vi "Elevator Control PID.vi"(8 "Settings":T2={"output range"={"output high"=1.0, "output low"=-0.75}, "min speed"=0.05, "homing speed"=0.05, "Position Max"=60.0, "PIDF gains"={"Kp"=0.2, "Ki"=0.0, "Kd"=0.2, "Kf"=0.0}, "gravity"=0.05, "Rate Limit in/sec"=30.0} {"Rate Limit in/sec" format="%#_13g"; "gravity" format="%#_13g"; "PIDF gains"."Kf" format="%.5f"; "PIDF gains"."Kd" format="%.3f"; "PIDF gains"."Ki" format="%.3f"; "PIDF gains"."Kp" format="%.3f"; "Position Max" format="%#_13g"; "homing speed" format="%#_13g"; "min speed" format="%#_13g"; "output range"."output low" format="%.2f"; "output range"."output high" format="%.2f"}, 9 "Manual":bool, 10 "Setpoint":dbl, 11 "Controller In":T3={"Setpoint"=0.0, "Output"=0.0, "DriveMotor1"={"DeviceStatus"={"status"=FALSE, "code"=0, "source"=""}, "Type"=enum."PWM", "PWM"={"PWM Channel"=enum."Invalid", "DeadBand"={"Name"="", "maxPositivePwm"=0, "minPositivePwm"=0, "centerPwm"=0, "maxNegativePwm"=0, "minNegativePwm"=0, "angularRange"=0}}, "CAN"={"Device Number"=0, "SetOutput VI Ref"=variant(enum8{"Percent VBus", "Current", "Speed", "Position", "Voltage"} enum."Percent VBus"), "GetOutput VI Ref"=variant(refnum<k1> refnum), "Enable VI Ref"=variant(dbl 12.0), "Disable VI Ref"=variant(enum8{"Percent VBus", "Speed", "Position", "Slave", "Unchanged / Invalid"} enum."Percent VBus"), "Data"=variant(enum16{"Controller 1"} enum."Controller 1")}, "Invert"=FALSE, "DIO PWM"={"PWM \"Enable\" Channel"=enum."Invalid", "DIOChannel"=enum."Invalid", "PWM Rate"=0.0}}, "Encoder"={"DevStatus"={"status"=FALSE, "code"=0, "source"=""}, "EncoderIndex"=enum."Invalid", "CounterIndex"=enum."Invalid", "DistancePerCount"=1.0, "Decoding Type"=enum."4x"}, "DriveMotor2"={"DeviceStatus"={"status"=FALSE, "code"=0, "source"=""}, "Type"=enum."PWM", "PWM"={"PWM Channel"=enum."Invalid", "DeadBand"={"Name"="", "maxPositivePwm"=0, "minPositivePwm"=0, "centerPwm"=0, "maxNegativePwm"=0, "minNegativePwm"=0, "angularRange"=0}}, "CAN"={"Device Number"=0, "SetOutput VI Ref"=variant(enum8{"Percent VBus", "Current", "Speed", "Position", "Voltage"} enum."Percent VBus"), "GetOutput VI Ref"=variant(refnum<k1> refnum), "Enable VI Ref"=variant(dbl 12.0), "Disable VI Ref"=variant(enum8{"Percent VBus", "Speed", "Position", "Slave", "Unchanged / Invalid"} enum."Percent VBus"), "Data"=variant(enum16{"Controller 1"} enum."Controller 1")}, "Invert"=FALSE, "DIO PWM"={"PWM \"Enable\" Channel"=enum."Invalid", "DIOChannel"=enum."Invalid", "PWM Rate"=0.0}}, "Top SW"={"DevStatus"={"status"=FALSE, "code"=0, "source"=""}, "DIO Channel"=enum."Invalid"}, "Bottom SW"={"DevStatus"={"status"=FALSE, "code"=0, "source"=""}, "DIO Channel"=enum."Invalid"}, "Is Done Moving?"=FALSE}) -> (0 "Switches":T1, 1 "PID is Done?":bool, 2 "Graph Out":T14(graph), 3 "Controller out":T3={"Setpoint"=0.0, "Output"=0.0, "DriveMotor1"={"DeviceStatus"={"status"=FALSE, "code"=0, "source"=""}, "Type"=enum."PWM", "PWM"={"PWM Channel"=enum."Invalid", "DeadBand"={"Name"="", "maxPositivePwm"=0, "minPositivePwm"=0, "centerPwm"=0, "maxNegativePwm"=0, "minNegativePwm"=0, "angularRange"=0}}, "CAN"={"Device Number"=0, "SetOutput VI Ref"=variant(enum8{"Percent VBus", "Current", "Speed", "Position", "Voltage"} enum."Percent VBus"), "GetOutput VI Ref"=variant(refnum<k1> refnum), "Enable VI Ref"=variant(dbl 12.0), "Disable VI Ref"=variant(enum8{"Percent VBus", "Speed", "Position", "Slave", "Unchanged / Invalid"} enum."Percent VBus"), "Data"=variant(enum16{"Controller 1"} enum."Controller 1")}, "Invert"=FALSE, "DIO PWM"={"PWM \"Enable\" Channel"=enum."Invalid", "DIOChannel"=enum."Invalid", "PWM Rate"=0.0}}, "Encoder"={"DevStatus"={"status"=FALSE, "code"=0, "source"=""}, "EncoderIndex"=enum."Invalid", "CounterIndex"=enum."Invalid", "DistancePerCount"=1.0, "Decoding Type"=enum."4x"}, "DriveMotor2"={"DeviceStatus"={"status"=FALSE, "code"=0, "source"=""}, "Type"=enum."PWM", "PWM"={"PWM Channel"=enum."Invalid", "DeadBand"={"Name"="", "maxPositivePwm"=0, "minPositivePwm"=0, "centerPwm"=0, "maxNegativePwm"=0, "minNegativePwm"=0, "angularRange"=0}}, "CAN"={"Device Number"=0, "SetOutput VI Ref"=variant(enum8{"Percent VBus", "Current", "Speed", "Position", "Voltage"} enum."Percent VBus"), "GetOutput VI Ref"=variant(refnum<k1> refnum), "Enable VI Ref"=variant(dbl 12.0), "Disable VI Ref"=variant(enum8{"Percent VBus", "Speed", "Position", "Slave", "Unchanged / Invalid"} enum."Percent VBus"), "Data"=variant(enum16{"Controller 1"} enum."Controller 1")}, "Invert"=FALSE, "DIO PWM"={"PWM \"Enable\" Channel"=enum."Invalid", "DIOChannel"=enum."Invalid", "PWM Rate"=0.0}}, "Top SW"={"DevStatus"={"status"=FALSE, "code"=0, "source"=""}, "DIO Channel"=enum."Invalid"}, "Bottom SW"={"DevStatus"={"status"=FALSE, "code"=0, "source"=""}, "DIO Channel"=enum."Invalid"}, "Is Done Moving?"=FALSE})   [LabVIEW 2017]
uses:
  Typedef/Controller Data.ctl
  <vilib>/Rock Robotics/WPI/MotorControl/WPI_MotorControlDeviceRef.ctl
  <vilib>/Rock Robotics/WPI/MotorControl/WPI_MotorControlType.ctl
  <vilib>/Rock Robotics/SystemInterfaces/DIO/FPGA_DIOPWMChannel.ctl
  <vilib>/Rock Robotics/WPI/PWM/WPI_PWMDeadband.ctl
  <vilib>/Rock Robotics/SystemInterfaces/DIO/FPGA_DIOChannel.ctl
  <vilib>/Rock Robotics/WPI/Encoder/WPI_EncoderDevRef.ctl
  <vilib>/Rock Robotics/SystemInterfaces/Encoder/FPGA_EncoderIdx.ctl
  <vilib>/Rock Robotics/SystemInterfaces/Counter/FPGA_CounterCtrSystemIndex.ctl
  <vilib>/Rock Robotics/WPI/Encoder/WPI_EncoderType.ctl
  <vilib>/Rock Robotics/WPI/DigitalInput/WPI_DigitalInputDevRef.ctl
  Typedef/Elevator Settings.ctl
  Implementation/Elevator Position Global.vi
  <vilib>/addons/control/pid/pid.llb/PID Output Rate Limiter (DBL).vi
  <vilib>/addons/control/pid/NI_PID_pid.lvlib
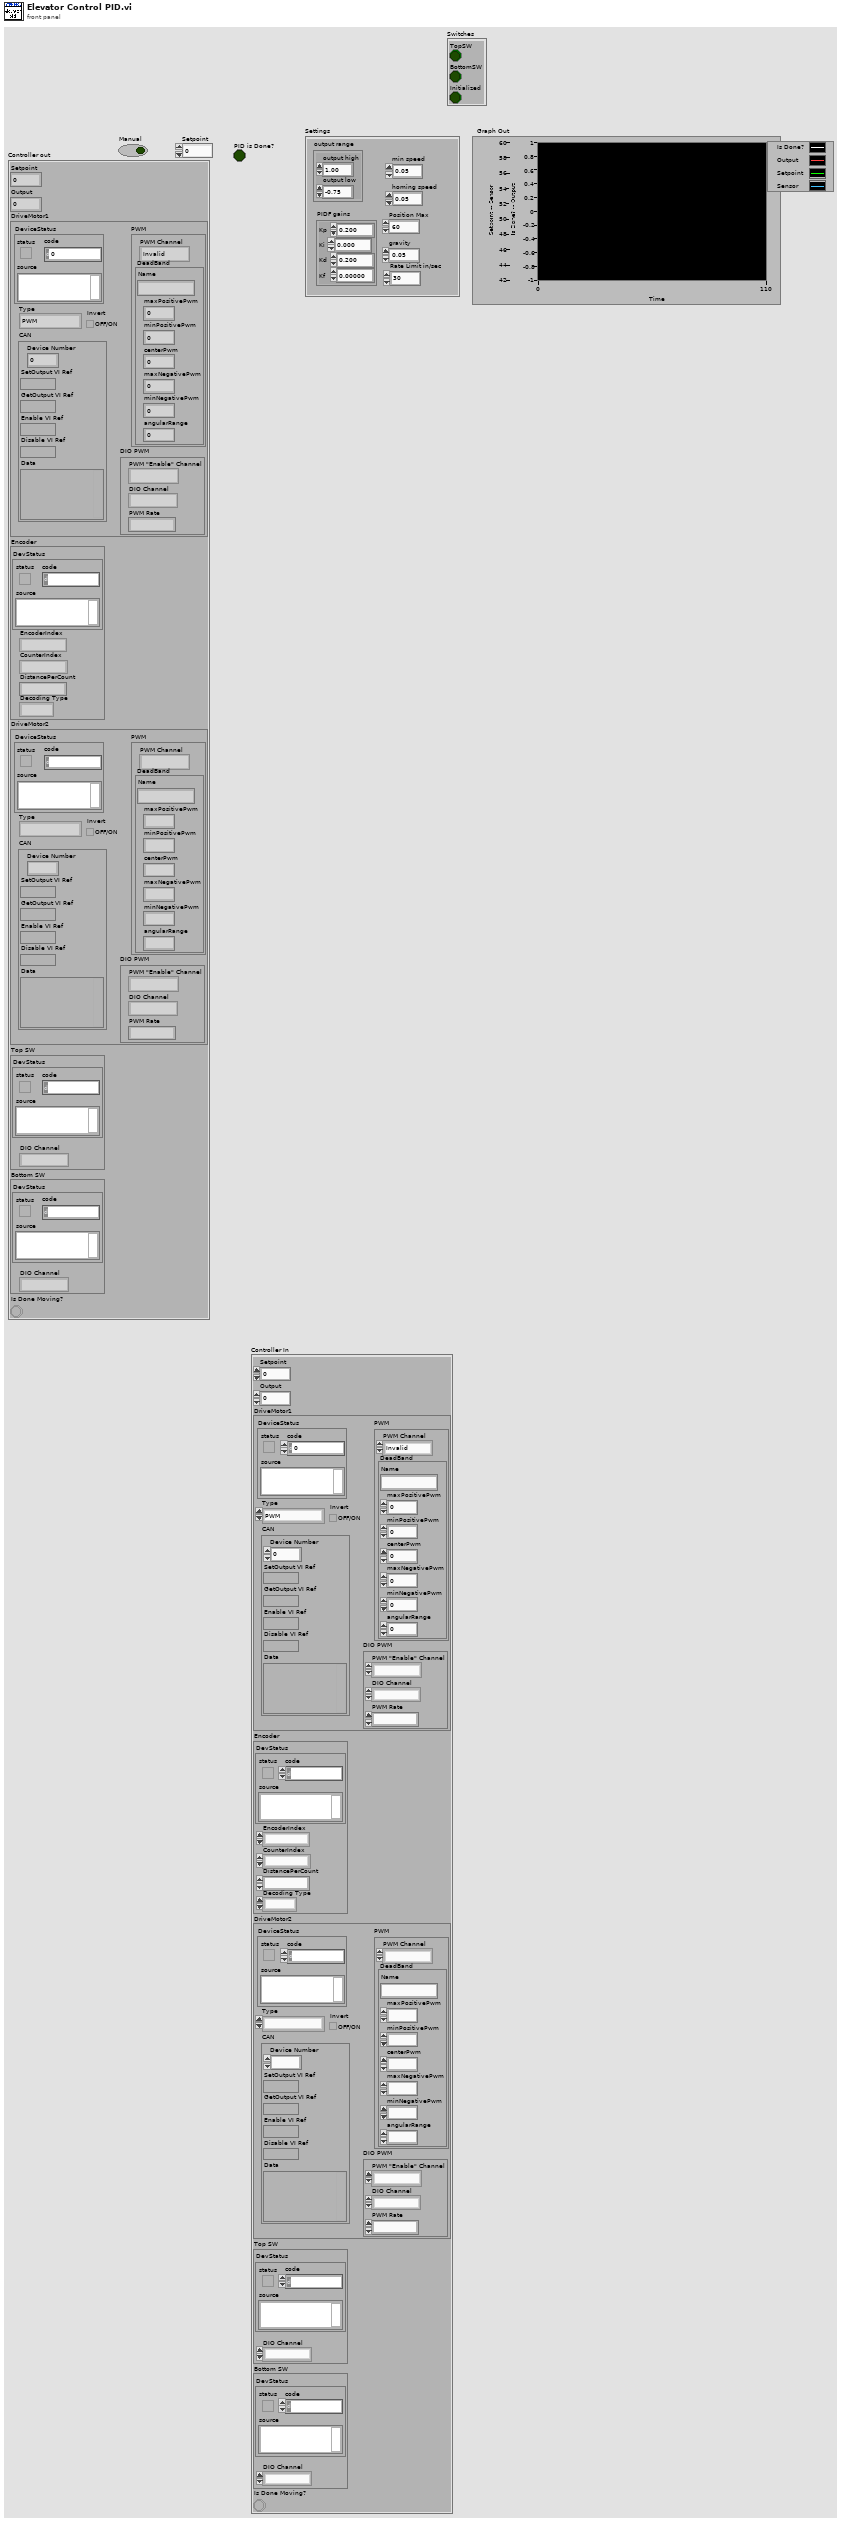
[diagram p1: front panel]
types:
  T1 = cluster{"TopSW":bool, "BottomSW":bool, "Initialized":bool}
  T2 = typedef "Elevator Settings.ctl" = cluster{"output range":cluster{"output high":dbl, "output low":dbl}, "min speed":dbl, "homing speed":dbl, "Position Max":dbl, "PIDF gains":cluster{"Kp":dbl, "Ki":dbl, "Kd":dbl, "Kf":dbl}, "gravity":dbl, "Rate Limit in/sec":dbl}
  T3 = typedef "Controller Data.ctl" = cluster{"Setpoint":dbl, "Output":dbl, "DriveMotor1":T4, "Encoder":T9, "DriveMotor2":T4, "Top SW":T13, "Bottom SW":T13, "Is Done Moving?":bool}
  T4 = typedef "WPI_MotorControlDeviceRef.ctl" = cluster{"DeviceStatus":errorcluster, "Type":T5, "PWM":cluster{"PWM Channel":T6, "DeadBand":T7}, "CAN":cluster{"Device Number":u8, "SetOutput VI Ref":variant, "GetOutput VI Ref":variant, "Enable VI Ref":variant, "Disable VI Ref":variant, "Data":variant}, "Invert":bool, "DIO PWM":cluster{"PWM \"Enable\" Channel":T6, "DIOChannel":T8, "PWM Rate":dbl}}
  T5 = typedef "WPI_MotorControlType.ctl" = enum16{"PWM", "CAN", "DIO PWM"}
  T6 = typedef "FPGA_DIOPWMChannel.ctl" = enum8{"PWM 0", "PWM 1", "PWM 2", "PWM 3", "PWM 4", "PWM 5", "PWM 6", "PWM 7", "PWM 8", "PWM 9", "PWM MXP 0", "PWM MXP 1", "PWM MXP 2", "PWM MXP 3", "PWM MXP 4", "PWM MXP 5", "PWM MXP 6", "PWM MXP 7", "PWM MXP 8", "PWM MXP 9", "Invalid"}
  T7 = typedef "WPI_PWMDeadband.ctl" = cluster{"Name":string, "maxPositivePwm":i32, "minPositivePwm":i32, "centerPwm":i32, "maxNegativePwm":i32, "minNegativePwm":i32, "angularRange":u16}
  T8 = typedef "FPGA_DIOChannel.ctl" = enum8{"DIO 0", "DIO 1", "DIO 2", "DIO 3", "DIO 4", "DIO 5", "DIO 6", "DIO 7", "DIO 8", "DIO 9", "DIO MXP 0", "DIO MXP 1", "DIO MXP 2", "DIO MXP 3", "DIO MXP 4", "DIO MXP 5", "DIO MXP 6", "DIO MXP 7", "DIO MXP 8", "DIO MXP 9", "DIO MXP 10", "DIO MXP 11", "DIO MXP 12", "DIO MXP 13", "DIO MXP 14", "DIO MXP 15", "SPI Port CS1", "SPI Port CS2", "SPI Port CS3", "SPI Port MISO", "SPI Port MOSI", "Invalid"}
  T9 = typedef "WPI_EncoderDevRef.ctl" = cluster{"DevStatus":errorcluster, "EncoderIndex":T10, "CounterIndex":T11, "DistancePerCount":dbl, "Decoding Type":T12}
  T10 = typedef "FPGA_EncoderIdx.ctl" = enum8{"Enc 0", "Enc 1", "Enc 2", "Enc 3", "Enc 4", "Enc 5", "Enc 6", "Enc 7", "Invalid"}
  T11 = typedef "FPGA_CounterCtrSystemIndex.ctl" = enum8{"Ctr 0", "Ctr 1", "Ctr 2", "Ctr 3", "Ctr 4", "Ctr 5", "Ctr 6", "Ctr 7", "Invalid"}
  T12 = typedef "WPI_EncoderType.ctl" = enum16{"1x", "2x", "4x"}
  T13 = typedef "WPI_DigitalInputDevRef.ctl" = cluster{"DevStatus":errorcluster, "DIO Channel":T8}
  T14 = cluster{i16, dbl, "Setpoint":dbl, "Distance":dbl}
  T15 = cluster{i16, dbl, "Position Max":dbl, "Distance":dbl}
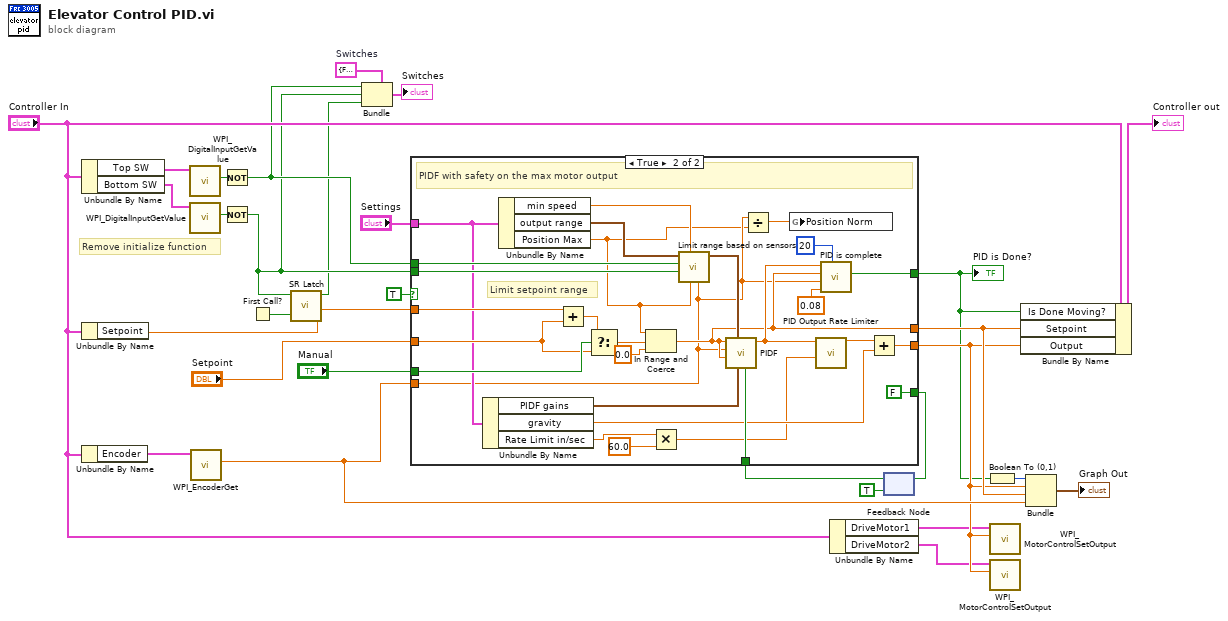
[diagram p0: block diagram]
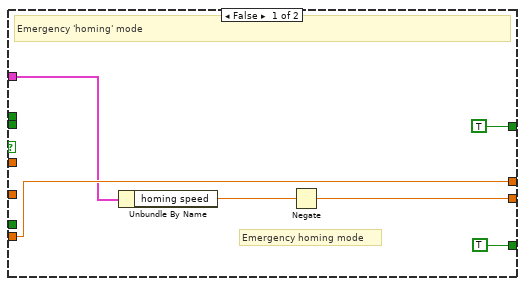
[diagram p2: hidden frame]
diagram:
  w6 = T1 {"TopSW"=FALSE, "BottomSW"=FALSE, "Initialized"=FALSE}  # Switches
  # "Remove initialize function"
  n1 = Unbundle By Name("Controller In") -> ("Top SW"=w20:T13, "Bottom SW"=w21:T13)
  n2 = Unbundle By Name("Controller In") -> ("Setpoint"=w17:dbl)
  n3 = Unbundle By Name("Controller In") -> ("Encoder"=w24:T9)
  n4 = call <vilib>:"WPI_DigitalInputGetValue.vi"("DigitalInputDevRef"=w20) -> ("Value"=w22:bool)  [unwired: 8 in, 2 out]
  n5 = call <vilib>:"WPI_DigitalInputGetValue.vi"("DigitalInputDevRef"=w21) -> ("Value"=w23:bool)  [unwired: 8 in, 2 out]
  n6 = call <vilib>:"WPI_EncoderGet.vi"("EncoderDevRef"=w24) -> ("Distance"=w28:dbl)  [unwired: 5 in, 5 out]
  n7 = Not(x=w22) -> (.not. x?=w5:bool)
  n8 = Not(x=w23) -> (.not. x?=w4:bool)
  n9 = First Call?() -> (First Call?: T/F=w9:bool)
  n10 = call "SR Latch.vi"("Reset"=w9, "Value"=w4) -> ("Latched"=w3:bool)  [unwired: 7 in]
  n11 = Bundle(cluster=w6, "TopSW"=w5, "BottomSW"=w4, "Initialized"=w3) -> (→"Switches":T1)
  n12 = Unbundle By Name("Controller In") -> ("DriveMotor1"=w18:T4, "DriveMotor2"=w19:T4)
  n13 = feedback #1(TRUE ("Reinitialize")) -> (w15:bool)
  n14 = case shown="True" TRUE {
    tunnel: "Setpoint" -> [_ w52]
    tunnel: [w33 w62] -> w25
    tunnel: w5 -> [_ w61]
    tunnel: w4 -> [_ w60]
    tunnel: [w32 w40] -> w26
    tunnel: [TRUE ("PID is Done?") w59] -> w7
    tunnel: [TRUE ("Reinitialize") FALSE ("Reinitialize?")] -> w14
    tunnel: w15 -> [_ w58]
    tunnel: "Manual" -> [_ w56]
    tunnel: w17 -> [_ w54]
    tunnel: w28 -> [w32 w38]
    tunnel: "Settings" -> [w31 w48]
    frame False {
      # "Emergency homing mode"
      # "Emergency 'homing' mode"
      n15 = Unbundle By Name(w31) -> ("homing speed"=w30:dbl)
      n16 = Negate(x=w30) -> (-x=w33:dbl)
    }
    frame True {
      # "Limit setpoint range"
      # "PIDF with safety on the max motor output"
      n17 = Unbundle By Name(w48) -> ("PIDF gains"=w47:cluster{"Kp":dbl, "Ki":dbl, "Kd":dbl, "Kf":dbl}, "gravity"=w46:dbl, "Rate Limit in/sec"=w43:dbl)
      n18 = Unbundle By Name(w48) -> ("min speed"=w50:dbl, "output range"=w49:cluster{"output high":dbl, "output low":dbl}, "Position Max"=w37:dbl)
      n19 = Add(x=w54, y=w52) -> (x+y=w55:dbl)
      n20 = Select(t=w55, s=w56, f=w52) -> (s? t:f=w51:dbl)
      n21 = In Range and Coerce(upper limit=w37, x=w51, lower limit=0.0) -> (coerced(x)=w40:dbl)  [unwired: 1 out]
      n22 = Multiply(x=w43, y=60.0 ("x")) -> (x*y=w42:dbl)
      n23 = call "Limit range based on sensors.vi"("Position"=w38, "Position Max"=w37, "min speed"=w50, "Bottom SW"=w60, "Top SW"=w61, "output range in"=w49) -> ("output range out"=w63:cluster{"output high":dbl, "output low":dbl})  [unwired: 5 in]
      n24 = call "PIDF.vi"("reinitialize? (F)"=w58, "PIDF gains"=w47, "output range"=w63, "Feedforward"=w40, "process variable"=w38, "setpoint"=w40) -> ("output"=w45:dbl)  [unwired: 3 in, 2 out]
      n25 = Divide(x=w38, y=w37) -> (x/y=w36:dbl)
      n26 = global write "Elevator Position Global.vi" "Position Norm"(w36) -> ()
      n27 = call-poly <vilib>:"PID Output Rate Limiter.vi"("output rate (EGU/min)"=w42, "input (controller output)"=w45) -> ("output"=w44:dbl)  [unwired: 6 in, 1 out]
      n28 = call "PID is complete.vi"("sample length"=20, "threshold"=0.08, "process variable"=w38, "setpoint"=w40, "PID Output"=w45) -> ("PID is Done?"=w59:bool)  [unwired: 5 in, 1 out]
      n29 = Add(x=w44, y=w46) -> (x+y=w62:dbl)
    }
  }
  "PID is Done?" <- w7
  n30 = feedback-in #1(w14) -> ()
  n31 = Boolean To (0,1)(Boolean=w7) -> (0, 1=w29:i16)
  n32 = call <vilib>:"WPI_MotorControlSetOutput.vi"("Output"=w25, "MotorControlDevRef"=w18) -> ()  [unwired: 7 in, 3 out]
  n33 = call <vilib>:"WPI_MotorControlSetOutput.vi"("Output"=w25, "MotorControlDevRef"=w19) -> ()  [unwired: 7 in, 3 out]
  n34 = Bundle By Name(cluster="Controller In", "Is Done Moving?"=w7, "Setpoint"=w26, "Output"=w25) -> (→"Controller out":T3)
  n35 = Bundle(w29, w25, "Position Max"=w26, "Distance"=w28) -> (→"Graph Out":T15)  [unwired: 1 in]
